vi "Create key line.vi"(8 "formatted value":string, 11 "key description":string) -> (3 "line":string)   [LabVIEW 2020, in "infolib.lvlib"]
doc: "Create a key line from description and value."
uses:
  infolib.lvlib
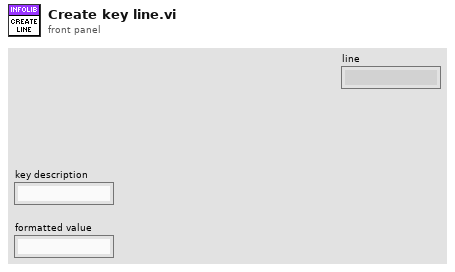
[diagram p1: front panel]
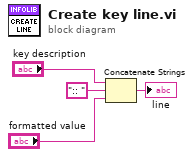
[diagram p0: block diagram]
diagram:
  n1 = Concatenate Strings("key description", ":: " ("string"), "formatted value") -> (→"line":string)
